vi "Add Waveforms from ListBox.vi"(6 "UI Refs":T2, 8 "error in":errorcluster, 9 "Wfm Ref LUT":variant, 10 "CD Settings in":T3 {"CD Task Dependency Ref" format="%.0x"; "CD Task Dependency" format="%.0x"}, 11 "Custom Device Ref in":T1 format="%.0x") -> (0 "error out":errorcluster, 1 "Wfm Ref LUT out":variant, 2 "CD Settings out":T3 {"CD Task Dependency Ref" format="%.0x"; "CD Task Dependency" format="%.0x"}, 3 "Custom Device Ref out":T1 format="%.0x")   [LabVIEW 2017, in "Waveform-Processing-Custom-Device System Explorer.lvlib"]
uses:
  Waveform-Processing-Custom-Device System Explorer.lvlib
  Shared/Custom Device Settings.ctl
  <vilib>/NI Veristand/Custom Device API/Custom Device Item Ref.ctl
  Types/UI Refs Ctl.ctl
  <vilib>/NI Veristand/Custom Device API/Custom Device Pointer.ctl
  <vilib>/NI VeriStand/Custom Device API/Custom Device API.lvlib
  NationalInstruments.VeriStand.SystemStorage
  Shared/Waveform-Processing-Custom-Device Shared.lvlib
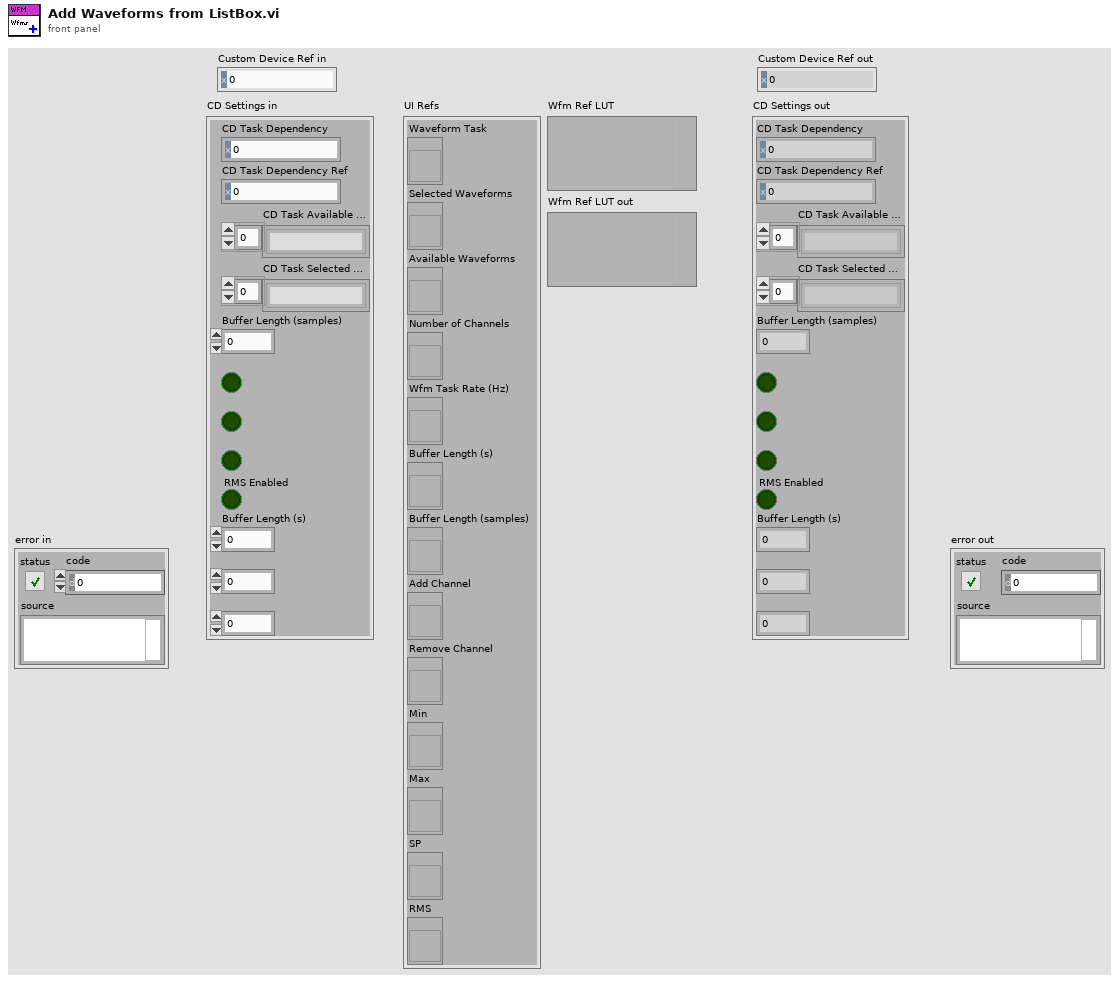
[diagram p1: front panel]
types:
  T1 = typedef "Custom Device API.lvlib/Custom Device Item Ref.ctl" = u64
  T2 = typedef "Waveform-Processing-Custom-Device Shared.lvlib/UI Refs Ctl.ctl" = cluster{"Waveform Task":refnum<vi>, "Selected Waveforms":refnum<vi>, "Available Waveforms":refnum<vi>, "Number of Channels":refnum<vi>, "Wfm Task Rate (Hz)":refnum<vi>, "Buffer Length (s)":refnum<vi>, "Buffer Length (samples)":refnum<vi>, "Add Channel":refnum<vi>, "Remove Channel":refnum<vi>, "Min":refnum<vi>, "Max":refnum<vi>, "SP":refnum<vi>, "RMS":refnum<vi>}
  T3 = typedef "Waveform-Processing-Custom-Device Shared.lvlib/Custom Device Settings.ctl" = cluster{"CD Task Dependency":T1, "CD Task Dependency Ref":T1, "CD Task Available Wfms":string[], "CD Task Selected Wfms":string[], "Buffer Length (samples)":u32, "Min Enabled":bool, "Max Enabled ":bool, "SP Enabled":bool, "RMS Enabled":bool, "Buffer Length (s)":dbl, "Task Rate":dbl, "Number of DAQ Chanels":u32}
  T4 = typedef "Custom Device API.lvlib/Custom Device Pointer.ctl" = refnum<k24>
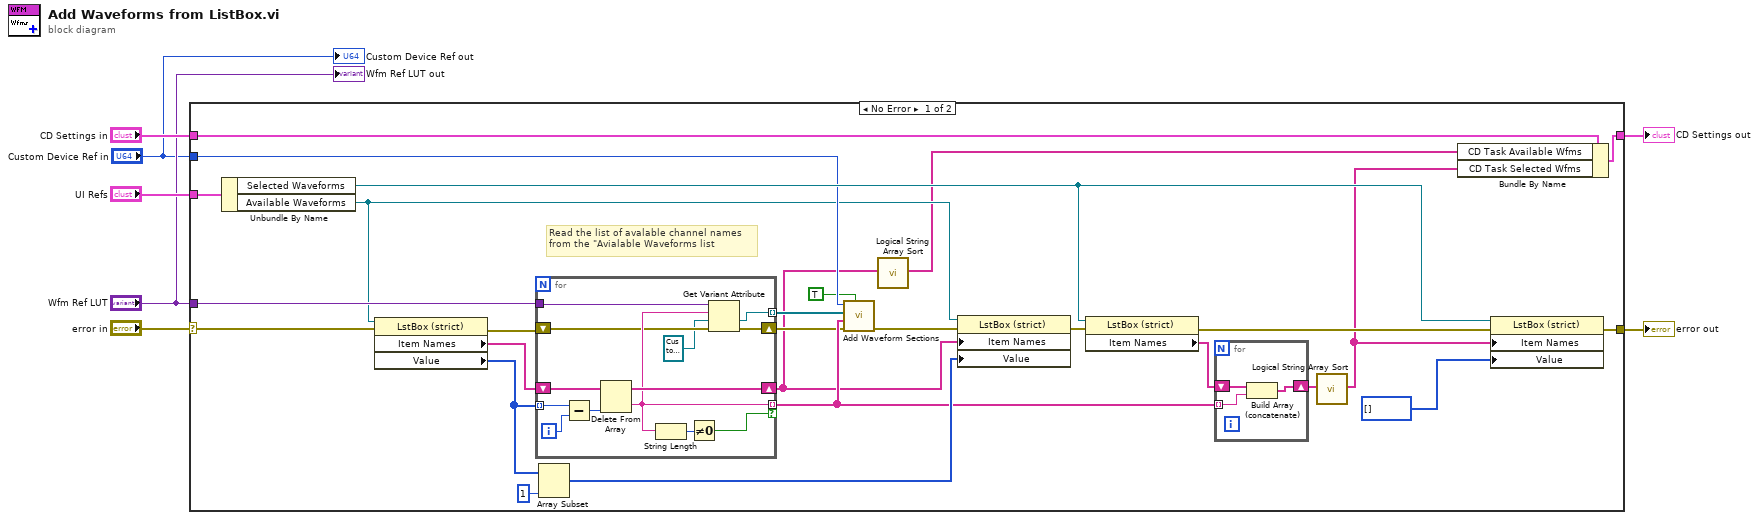
[diagram p0: block diagram]
diagram:
  n1 = case shown="No Error" "error in" {
    selector: "error in" -> [w23 w51]
    tunnel: [w31 w52] -> w7
    tunnel: "CD Settings in" -> [w30 w52]
    tunnel: [w18 w51] -> w5
    tunnel: "UI Refs" -> [w28 _]
    tunnel: "Wfm Ref LUT" -> [w25 _]
    tunnel: "Custom Device Ref in" -> [w24 _]
    frame No Error {
      # "Read the list of avalable channel names\nfrom the \"Avialable Waveforms list"
      n2 = Unbundle By Name(w28) -> ("Selected Waveforms"=w27:refnum<vi>, "Available Waveforms"=w22:refnum<vi>)
      n3 = property on="Property Node" class="LstBox (strict)"(reference=w22, error in=w23) -> (error out=w21:errorcluster, "Item Names"=w19:string[], "Value"=w20:i32[])  [unwired: 1 out]
      n4 = for {
        tunnel: w20 -> [w44] mode=indexing
        shift-right: [w46] -> w8
        shift-left: w19 -> [w47]
        tunnel: [w40] -> w14 mode=indexing if=w36
        tunnel: w25 -> [w41]
        shift-right: [w38] -> w13
        shift-left: w21 -> [w39]
        tunnel: [w37] -> w17 mode=indexing
        i -> [w45]
        n5 = Subtract(x=w44, y=w45) -> (x-y=w43:i32)
        n6 = Delete From Array(array=w47, index=w43) -> (deleted portion=w40:string, array with subset deleted=w46:string[])  [unwired: 1 in]
        n7 = String Length(string=w40) -> (length=w42:i32)
        n8 = Not Equal To 0?(x=w42) -> (x != 0?=w36:bool)
        n9 = Get Variant Attribute(Variant=w41, name=w40, default value (empty Variant)=T4 refnum ("Node Pointer"), error in=w39) -> (value=w37:T4, error out=w38:errorcluster)  [unwired: 2 out]
      }
      n10 = Array Subset(array=w20, length=1) -> (w33:i32[])  [unwired: 1 in]
      n11 = call "Add Waveform Sections.vi"("Names List"=TRUE, "Error In"=w13, "External Names"=w14, "Wfm Pointers"=w17, "CustomDevice Ref"=w24) -> ("Error Out"=w12:errorcluster)  [unwired: 5 in, 1 out]
      n12 = call "Logical String Array Sort.vi"("Unsorted List"=w8) -> ("Sorted List"=w9:string[])  [unwired: 18 in]
      n13 = property on="Property Node" class="LstBox (strict)"(reference=w22, error in=w12, "Item Names"=w8, "Value"=w33) -> (error out=w29:errorcluster)  [unwired: 1 out]
      n14 = property on="Property Node" class="LstBox (strict)"(reference=w27, error in=w29) -> (error out=w11:errorcluster, "Item Names"=w32:string[])  [unwired: 1 out]
      n15 = for {
        tunnel: w14 -> [w49] mode=indexing
        shift-right: [w48] -> w15
        shift-left: w32 -> [w50]
        n16 = Build Array (concatenate)(w50, w49) -> (w48:string[])
      }
      n17 = call "Logical String Array Sort.vi"("Unsorted List"=w15) -> ("Sorted List"=w10:string[])  [unwired: 18 in]
      n18 = Bundle By Name(cluster=w30, "CD Task Available Wfms"=w9, "CD Task Selected Wfms"=w10) -> (w31:T3)
      n19 = property on="Property Node" class="LstBox (strict)"(reference=w27, error in=w11, "Item Names"=w10, "Value"=i32[] [] ("Waveforms to Process")) -> (error out=w18:errorcluster)  [unwired: 1 out]
    }
    frame Error {
    }
  }
  "CD Settings out" <- w7
  "error out" <- w5
  "Custom Device Ref out" <- "Custom Device Ref in"
  "Wfm Ref LUT out" <- "Wfm Ref LUT"
